vi "RIO Page.vi"(8 "error in (no error)":errorcluster, 11 "Node Ptr":T1 format="%.0x") -> (0 "error out":errorcluster)   [LabVIEW 2017, in "Engine Simulation Toolkit System Explorer.lvlib"]
uses:
  Engine Simulation Toolkit System Explorer.lvlib
  <vilib>/NI Veristand/Custom Device API/Custom Device Item Ref.ctl
  <vilib>/NI Veristand/Custom Device Tools/Custom Device Utility Library/Search Direction.ctl
  Shared/Constants and GUIDs.vi
  <vilib>/NI Veristand/Custom Device Tools/Custom Device Utility Library/NI VeriStand - Search for Item by GUID.vi
  Shared/Properties.vi
  <vilib>/NI Veristand/Custom Device API/Get Item Property (Dependent File).vi
  <vilib>/NI Veristand/Custom Device API/Get Item Property (String).vi
  <vilib>/NI Veristand/Custom Device API/Custom Device API.lvlib
  Shared/Engine Simulation Toolkit Shared.lvlib
  <vilib>/NI Veristand/Custom Device Tools/Custom Device Utility Library/Custom Device Utility Library.lvlib
panel:
  out "Bitfile Path":string
  out "Version of EST in Bitfile":string
  out "RIO Device Address":string
  in  "Header":cluster{"Section Name":string}={"Section Name"="RIO Device Configuration"}
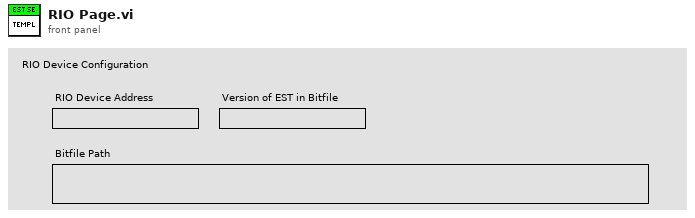
[diagram p1: front panel]
types:
  T1 = typedef "Custom Device API.lvlib/Custom Device Item Ref.ctl" = u64
  T2 = typedef "Custom Device Utility Library.lvlib/Search Direction.ctl" = enum16{"Down", "Up"}
  T3 = typedef "Custom Device API.lvlib/Custom Device Item Info.ctl" = cluster{"Name":string, "Is Channel":bool, "GUID":string, "Is Waveform":bool}
  T4 = typedef "Custom Device API.lvlib/Custom Device Commands.ctl" = enum16{"Default", "Item renamed", "Shutdown", "Dynamic button pressed"}
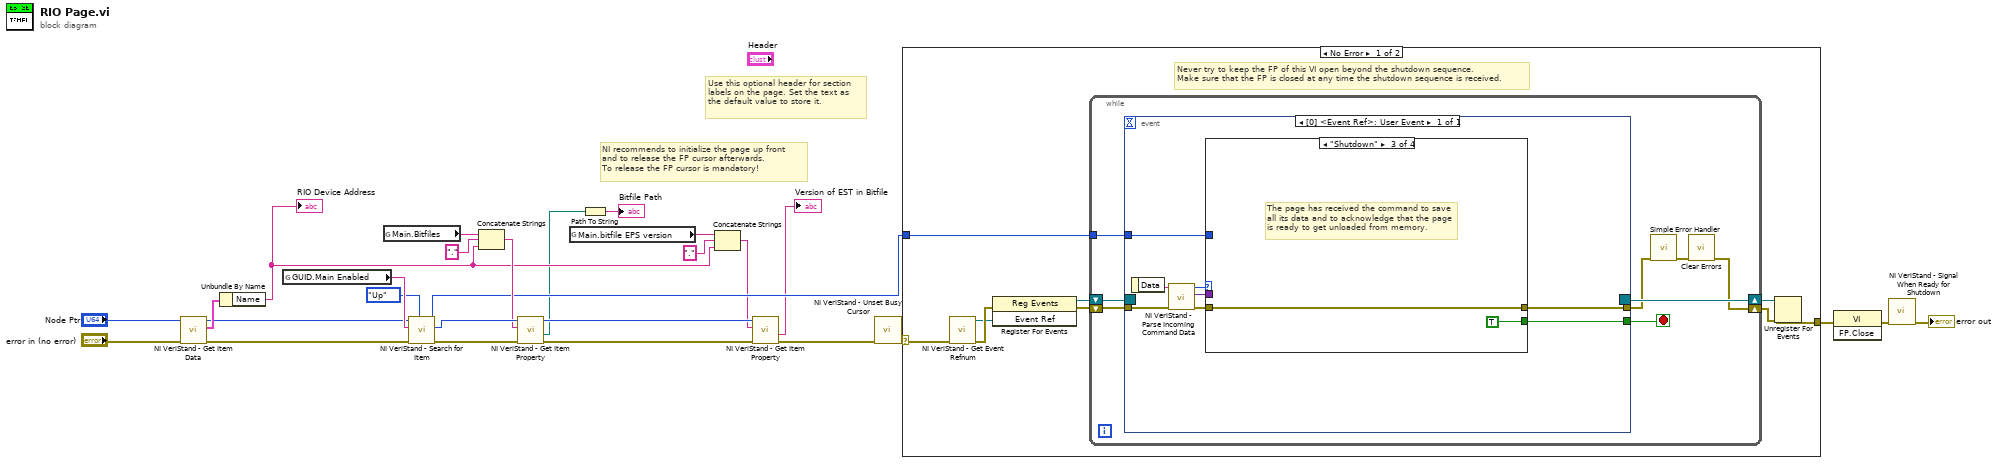
[diagram p0: block diagram]
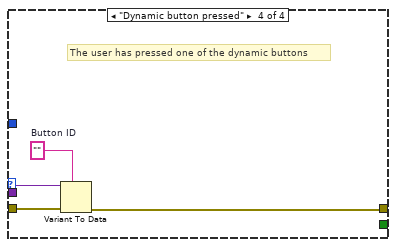
[diagram p4: hidden frame]
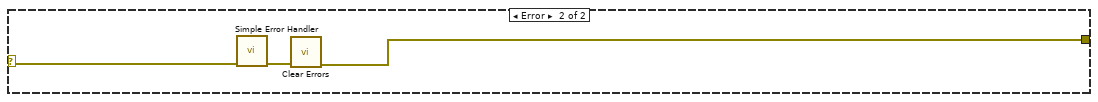
[diagram p5: hidden frame]
diagram:
  # "Use this optional header for section labels on the page. Set the text as the default value to store it."
  # "NI recommends to initialize the page up front\nand to release the FP cursor afterwards.\nTo release the FP cursor is mandatory!"
  n1 = call <vilib>:"NI VeriStand - Get Item Data.vi"("error in (no error)"="error in (no error)", "Item Ref in"="Node Ptr") -> ("error out"=w20:errorcluster, "Item Info"=w21:T3, "Item Ref out"=w18:T1)  [unwired: 6 in, 1 out]
  n2 = Unbundle By Name(w21) -> ("Name"=w5:string)
  "RIO Device Address" <- w5
  n3 = global read "Constants and GUIDs.vi" "GUID.Main Enabled"() -> (w19:string)
  n4 = global read "Properties.vi" "Main.Bitfiles"() -> (w15:string)
  n5 = call-poly <vilib>:"NI VeriStand - Search for Item.vi"("Direction (Down)"=Search_Direction."Up", "error in"=w20, "Item GUID"=w19, "Section Ref in"=w18) -> ("error out"=w17:errorcluster, "Item Ref"=w16:T1, "Section Ref out"=w11:T1)  [unwired: 4 in, 1 out]
  n6 = Concatenate Strings(w15, "." ("string"), w5) -> (w13:string)
  n7 = call-poly <vilib>:"NI VeriStand - Get Item Property.vi"("error in (no error)"=w17, "Property Name"=w13, "Item Ref in"=w16) -> ("error out"=w12:errorcluster, "Path"=w1:path, "Item Ref out"=w9:T1)  [unwired: 4 in, 2 out]
  n8 = global read "Properties.vi" "Main.bitfile EPS version"() -> (w7:string)
  n9 = Path To String(path=w1) -> (string=→"Bitfile Path":string)
  n10 = Concatenate Strings(w7, "." ("string"), w5) -> (w6:string)
  n11 = call-poly <vilib>:"NI VeriStand - Get Item Property.vi"("error in (no error)"=w12, "Property Name"=w6, "Item Ref in"=w9) -> ("error out"=w10:errorcluster, "Value"=→"Version of EST in Bitfile":string)  [unwired: 5 in, 2 out]
  n12 = call <vilib>:"NI VeriStand - Unset Busy Cursor.vi"("error in (no error)"=w10) -> ("error out"=w24:errorcluster)  [unwired: 10 out]
  n13 = case shown="No Error" w24 {
    selector: w24 -> [w29 w63]
    tunnel: [w33 w61] -> w27
    tunnel: w11 -> [w28 _]
    frame No Error {
      # "Never try to keep the FP of this VI open beyond the shutdown sequence.\nMake sure that the FP is closed at any time the shutdown sequence is received."
      n14 = call <vilib>:"NI VeriStand - Get Event Refnum.vi"("error in (no error)"=w29) -> ("error out"=w36:errorcluster, "Event Ref"=w32:refnum<user-event>)  [unwired: 9 out]
      n15 = register-events(error in=w36, w32) -> (reference out=w30:refnum<event-registration>, error out=w31:errorcluster)  [unwired: 1 in]
      n16 = while {
        shift-right: [w38] -> w34
        shift-left: w31 -> [w43]
        shift-right: [w44] -> w35
        shift-left: w30 -> [w42]
        tunnel: w28 -> [w37]
        stop <- w41 stop-if-true
        n17 = event shown="[0] <Event Ref>: User Event" {
          selector: w42 -> [_]
          dyn-events: [_] -> w44
          timeout: _ -> [_]
          tunnel: w43 -> [w52]
          tunnel: [w48] -> w41
          tunnel: [w47] -> w40
          tunnel: w37 -> [w45]
          event User Event {
            n18 = event-data() -> ("Data"=w51:string)  [unwired: 1 out]
            n19 = call <vilib>:"NI VeriStand - Parse Incoming Command Data.vi"("error in (no error)"=w52, "Incoming data"=w51) -> ("error out"=w50:errorcluster, "Outgoing data"=w46:variant, "Action"=w49:T4)  [unwired: 7 out]
            n20 = case shown="\"Shutdown\"" w49 {
              tunnel: w50 -> [w53 w54 w55 w60]
              tunnel: [_ _ TRUE _] -> w48
              tunnel: [w53 w54 w55 w57] -> w47
              tunnel: w46 -> [_ _ _ w59]
              tunnel: w45 -> [_ _ _ _]
              frame "Default", Default {
              }
              frame "Item renamed" {
              }
              frame "Shutdown" {
                # "The page has received the command to save all its data and to acknowledge that the page is ready to get unloaded from memory."
              }
              frame "Dynamic button pressed" {
                w58 = ""  # Button ID
                # "The user has pressed one of the dynamic buttons"
                n21 = Variant To Data(error in=w60, type=w58, Variant=w59) -> (error out=w57:errorcluster)  [unwired: 1 out]
              }
            }
          }
        }
        n22 = call <vilib>:"Simple Error Handler.vi"("error in (no error)"=w40) -> ("error out"=w39:errorcluster)  [unwired: 1 in, 7 out]
        n23 = call <vilib>:"Clear Errors.vi"("error in (no error)"=w39) -> ("error out"=w38:errorcluster)  [unwired: 1 in, 5 out]
      }
      n24 = Unregister For Events(event registration refnum=w35, error in=w34) -> (error out=w33:errorcluster)
    }
    frame Error {
      n25 = call <vilib>:"Simple Error Handler.vi"("error in (no error)"=w63) -> ("error out"=w62:errorcluster)  [unwired: 1 in, 7 out]
      n26 = call <vilib>:"Clear Errors.vi"("error in (no error)"=w62) -> ("error out"=w61:errorcluster)  [unwired: 1 in, 5 out]
    }
  }
  n27 = invoke class="VI" method="FP.Close"(error in=w27) -> (error out=w26:errorcluster)  [unwired: 2 in, 2 out]
  n28 = call <vilib>:"NI VeriStand - Signal When Ready for Shutdown.vi"("error in (no error)"=w26) -> ("error out"=→"error out":errorcluster)  [unwired: 10 out]
